vi "SignalGenerator_2.vi"(10 "Phase":fxp<+,64,64>[](array[numeric])=[0.0, 0.0], 11 "reset":bool) -> (1 "Sine out":fxp<+/-,16,0>[](array[numeric]), 2 "Cosine out":fxp<+/-,16,0>[](array[numeric]))   [LabVIEW 2013]
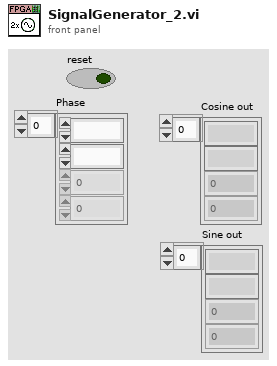
[diagram p1: front panel]
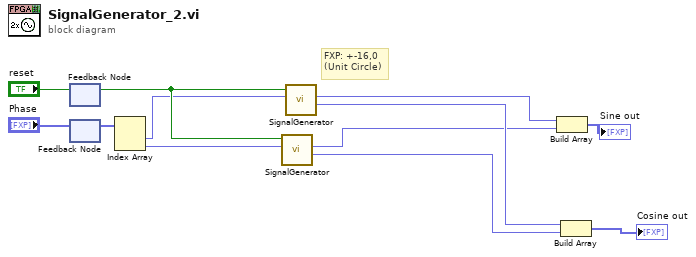
[diagram p0: block diagram]
diagram:
  # "FXP: +-16,0\n(Unit Circle)"
  n1 = feedback #1() -> (w6:bool)  [unwired: 1 in]
  n2 = feedback-in #1("reset") -> ()
  n3 = feedback #2() -> (w8:fxp<+,64,64>[])  [unwired: 1 in]
  n4 = feedback-in #2("Phase") -> ()
  n5 = Index Array(array=w8) -> (element #1=w5:fxp<+,64,64>, element #2=w10:fxp<+,64,64>)  [unwired: 2 in]
  n6 = call "SignalGenerator.vi"("phase"=w10, "Reset"=w6) -> ("Cos"=w1:fxp<+/-,16,0>, "Sin"=w2:fxp<+/-,16,0>)  [unwired: 7 in, 1 out]
  n7 = call "SignalGenerator.vi"("phase"=w5, "Reset"=w6) -> ("Cos"=w3:fxp<+/-,16,0>, "Sin"=w4:fxp<+/-,16,0>)  [unwired: 7 in, 1 out]
  n8 = Build Array(w4, w2) -> (→"Sine out":fxp<+/-,16,0>[])
  n9 = Build Array(w3, w1) -> (→"Cosine out":fxp<+/-,16,0>[])
